vi "for loop.vi"() -> ()   [LabVIEW 2011]
panel:
  out "Array":dbl[](array[numeric])
  out "Factorial":dbl
  in  "Number":dbl
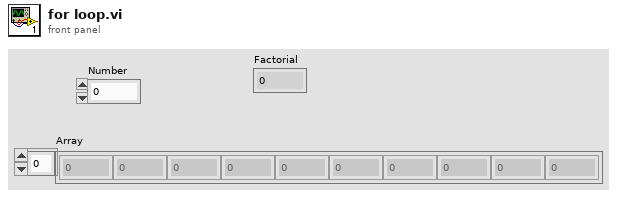
[diagram p1: front panel]
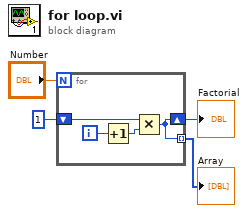
[diagram p0: block diagram]
diagram:
  n1 = for {
    N: "Number" -> [_]
    tunnel: [w5] -> w1 mode=indexing
    shift-right: [w5] -> w2
    shift-left: 1 -> [w6]
    i -> [w8]
    n2 = Increment(x=w8) -> (x+1=w7:i32)
    n3 = Multiply(x=w6, y=w7) -> (x*y=w5:i32)
  }
  "Factorial" <- w2
  "Array" <- w1
